vi "IAStateToGameNavigationDefensive.vi"(8 "error in (no error)":errorcluster, 10 "our_robots":T1[](array[typedef]), 11 "Game in":refnum<class "Game.lvclass">) -> (0 "error out":errorcluster, 3 "Game out":refnum<class "Game.lvclass">)   [LabVIEW 2018, in "Game.lvclass"]
uses:
  Game.lvclass
  Vision_class/Old vision/Controls/AI Robot.ctl
  Vision_class/Old vision/Controls/Functions Enum.ctl
  Vision_class/Old vision/Controls/AttackerStates.ctl
  Vision_class/Old vision/Controls/PathDests.ctl
  Vision_class/Old vision/Controls/PathDest.ctl
  Game.lvclass/Game.ctl
  Team_class/Team.lvclass/Team.ctl
  Robot_class/Robot.lvclass/Robot.ctl
  Robot_class/Write v_norm.vi
  Robot_class/Write v_tang.vi
  Robot_class/Write v_ang.vi
  Robot_class/Write vx_desired.vi
  Robot_class/Write vy_desired.vi
  Read DefensiveTeam.vi
  Team_class/Read RobotRef.vi
  Team_class/Write RobotRef.vi
  Write DefensiveTeam.vi
  Ally_class/Ally.lvclass
  C:/Users/Guilherme Moreira/OneDrive/Dokumente/SSL_AI_nicolas/SSL_AI/Team_class/Team.lvclass
  Robot_class/Robot.lvclass
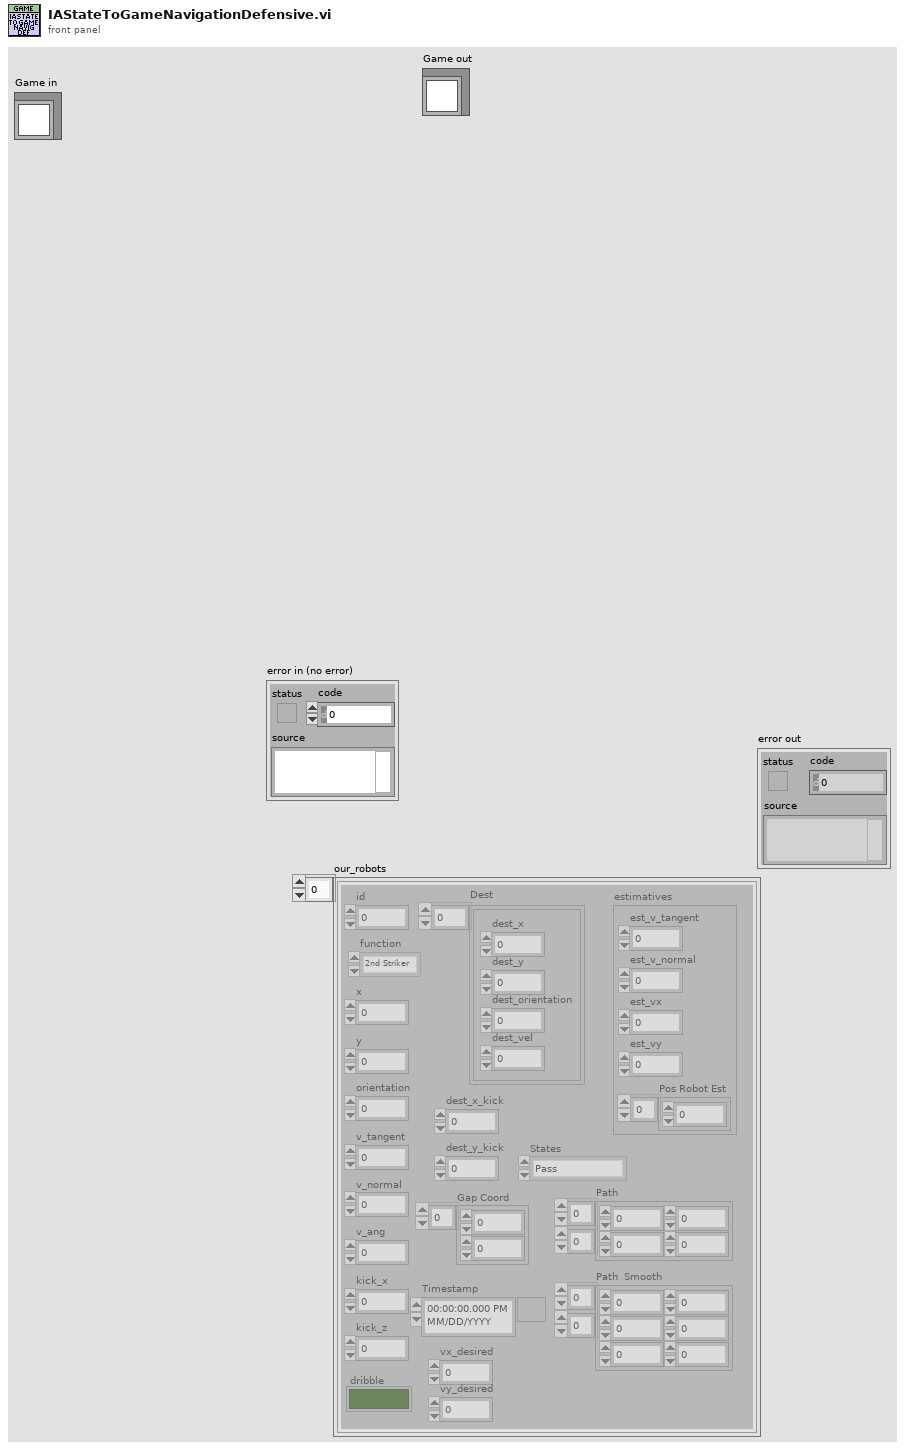
[diagram p1: front panel]
types:
  T1 = typedef "AI Robot.ctl" = cluster{"id":u32, "function":T2, "x":dbl, "y":dbl, "orientation":dbl, "v_tangent":dbl, "v_normal":dbl, "v_ang":dbl, "kick_x":dbl, "kick_z":dbl, "dribble":bool, "Timestamp":timestamp, "estimatives":cluster{"est_v_tangent":dbl, "est_v_normal":dbl, "est_vx":dbl, "est_vy":dbl, "Pos Robot Est":dbl[]}, "dest_x_kick":dbl, "dest_y_kick":dbl, "Gap Coord":dbl[], "States":T3, "Path ":dbl[][], "Path  Smooth":dbl[][], "Dest":T4, "vx_desired":dbl, "vy_desired":dbl}
  T2 = typedef "Functions Enum.ctl" = enum16{"2nd Striker", "Attacker", "Goalie", "Defender", "Striker", "Goto 0", "Dummy", "Kicker", "ZigZag 0", "ZigZag 1", "ZigZag 2", "ZigZag 3", "ZigZag 4", "ZigZag 5", "ZigZag 6", "ZigZag 7", "ZigZag 8", ""}
  T3 = typedef "AttackerStates.ctl" = enum16{"Pass", "GoToTangent", "BallGetting", "GoToKick", ""}
  T4 = typedef "PathDests.ctl" = T5[]
  T5 = typedef "PathDest.ctl" = cluster{"dest_x":dbl, "dest_y":dbl, "dest_orientation":dbl, "dest_vel":dbl}
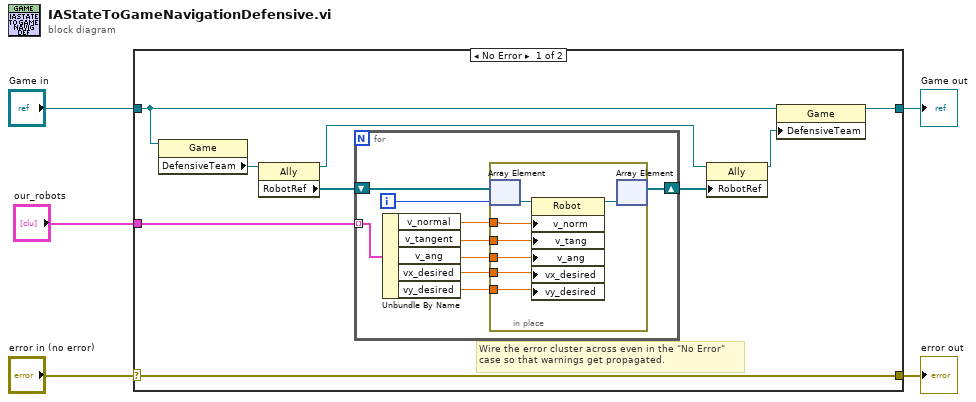
[diagram p0: block diagram]
diagram:
  n1 = case shown="No Error" "error in (no error)" {
    selector: "error in (no error)" -> [w14 w32]
    tunnel: [w14 w32] -> w4
    tunnel: [w13 w31] -> w2
    tunnel: "Game in" -> [w12 w31]
    tunnel: "our_robots" -> [w9 _]
    frame No Error {
      # "Wire the error cluster across even in the \"No Error\"\ncase so that warnings get propagated."
      n2 = property class="Game"(reference=w12) -> ("DefensiveTeam"=w11:refnum<class "Ally.lvclass">)  [unwired: 1 in, 2 out]
      n3 = property class="Ally"(reference=w11) -> (reference out=w6:refnum<class "Ally.lvclass">, "RobotRef"=w10:refnum<class "Robot.lvclass">[])  [unwired: 1 in, 1 out]
      n4 = for {
        tunnel: w9 -> [w21] mode=indexing
        shift-right: [w20] -> w7
        shift-left: w10 -> [w22]
        i -> [w23]
        n5 = Unbundle By Name(w21) -> ("v_normal"=w19:dbl, "v_tangent"=w18:dbl, "v_ang"=w17:dbl, "vx_desired"=w16:dbl, "vy_desired"=w15:dbl)
        n6 = in-place {
          in-place-border: w19 -> [w28]
          in-place-border: w18 -> [w27]
          in-place-border: w17 -> [w26]
          in-place-border: w16 -> [w25]
          in-place-border: w15 -> [w24]
          n7 = in-place-array #1(w22, w23) -> (w30:refnum<class "Robot.lvclass">)
          n8 = property class="Robot"(reference=w30, "v_norm"=w28, "v_tang"=w27, "v_ang"=w26, "vx_desired"=w25, "vy_desired"=w24) -> (reference out=w29:refnum<class "Robot.lvclass">)  [unwired: 1 in, 1 out]
          n9 = in-place-array #1(w29) -> (w20:refnum<class "Robot.lvclass">[])  [unwired: 1 out]
        }
      }
      n10 = property class="Ally"(reference=w6, "RobotRef"=w7) -> (reference out=w8:refnum<class "Ally.lvclass">)  [unwired: 1 in, 1 out]
      n11 = property class="Game"(reference=w12, "DefensiveTeam"=w8) -> (reference out=w13:refnum<class "Game.lvclass">)  [unwired: 1 in, 1 out]
    }
    frame Error {
    }
  }
  "error out" <- w4
  "Game out" <- w2
